vi "Joystick Get Values.vi"(8 "error in (no error)":errorcluster, 11 "Joystick":T1) -> (0 "error out":errorcluster, 1 "Buttons":bool[](array[boolean]), 2 "Axes":dbl[](array[numeric]), 3 "Joystick":T1, 4 "POVs":u8[](array[numeric]), 5 "Touchpads":T2(array[cluster]))   [LabVIEW 2026, in "MrcLib.lvlib"]
doc: "Returns button and scaled axis information for a joystick that you specify."
uses:
  MrcLib.lvlib
  <vilib>/Rock Robotics/WPI/Joystick/WPI_JoystickDeviceEnum.ctl
panel:
  in  "Scaler":i16=32767
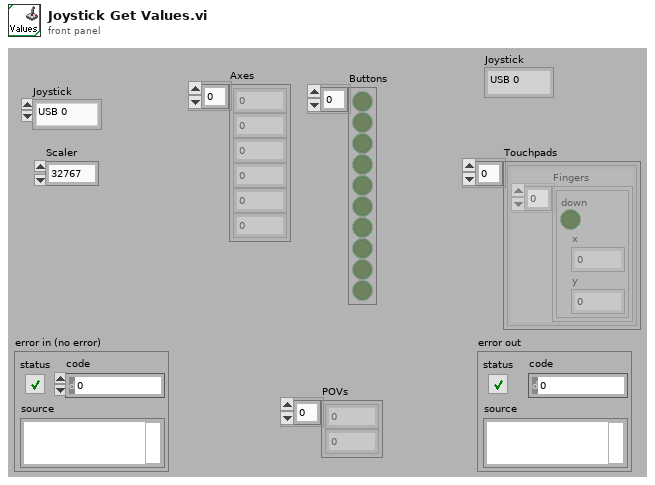
[diagram p1: front panel]
types:
  T1 = typedef "WPI_JoystickDeviceEnum.ctl" = enum16{"USB 0", "USB 1", "USB 2", "USB 3", "USB 4", "USB 5"}
  T2 = cluster{"Fingers":cluster{"down":bool, "x":u16, "y":u16}[]}[]
  T3 = cluster{cluster{"down":bool, "x":u16, "y":u16}[]}
  T4 = typedef "MrcLib.lvlib/MRC_Joysticks.ctl" = cluster{"count":u8, "dummy":cluster{i8, i8, i8, i8, i8, i8, i8}, "joystick 0":cluster{"availablePovs":u8, "povs":cluster{"pov 0":u8, "pov 1":u8, "pov 2":u8, "pov 3":u8, "pov 4":u8, "pov 5":u8, "pov 6":u8, "pov 7":u8}, "availableAxes":u16, "axes":cluster{"axis 0":i16, "axis 1":i16, "axis 2":i16, "axis 3":i16, "axis 4":i16, "axis 5":i16, "axis 6":i16, "axis 7":i16, "axis 8":i16, "axis 9":i16, "axis 10":i16, "axis 11":i16}, "availableButtons":u64, "buttons":u64, "touchPads":cluster{"touchPadCount":u8, "touchpad 1":cluster{"count":u8, "finger 1":cluster{"down":u8, "x":u16, "y":u16}, "finger 2":cluster{"down":u8, "x":u16, "y":u16}}, "touchpad 2":cluster{"count":u8, "finger 1":cluster{"down":u8, "x":u16, "y":u16}, "finger 2":cluster{"down":u8, "x":u16, "y":u16}}}}, "joystick 1":cluster{"availablePovs":u8, "povs":cluster{"pov 0":u8, "pov 1":u8, "pov 2":u8, "pov 3":u8, "pov 4":u8, "pov 5":u8, "pov 6":u8, "pov 7":u8}, "availableAxes":u16, "axes":cluster{"axis 0":i16, "axis 1":i16, "axis 2":i16, "axis 3":i16, "axis 4":i16, "axis 5":i16, "axis 6":i16, "axis 7":i16, "axis 8":i16, "axis 9":i16, "axis 10":i16, "axis 11":i16}, "availableButtons":u64, "buttons":u64, "touchPads":cluster{"touchPadCount":u8, "touchpad 1":cluster{"count":u8, "finger 1":cluster{"down":u8, "x":u16, "y":u16}, "finger 2":cluster{"down":u8, "x":u16, "y":u16}}, "touchpad 2":cluster{"count":u8, "finger 1":cluster{"down":u8, "x":u16, "y":u16}, "finger 2":cluster{"down":u8, "x":u16, "y":u16}}}}, "joystick 2":cluster{"availablePovs":u8, "povs":cluster{"pov 0":u8, "pov 1":u8, "pov 2":u8, "pov 3":u8, "pov 4":u8, "pov 5":u8, "pov 6":u8, "pov 7":u8}, "availableAxes":u16, "axes":cluster{"axis 0":i16, "axis 1":i16, "axis 2":i16, "axis 3":i16, "axis 4":i16, "axis 5":i16, "axis 6":i16, "axis 7":i16, "axis 8":i16, "axis 9":i16, "axis 10":i16, "axis 11":i16}, "availableButtons":u64, "buttons":u64, "touchPads":cluster{"touchPadCount":u8, "touchpad 1":cluster{"count":u8, "finger 1":cluster{"down":u8, "x":u16, "y":u16}, "finger 2":cluster{"down":u8, "x":u16, "y":u16}}, "touchpad 2":cluster{"count":u8, "finger 1":cluster{"down":u8, "x":u16, "y":u16}, "finger 2":cluster{"down":u8, "x":u16, "y":u16}}}}, "joystick 3":cluster{"availablePovs":u8, "povs":cluster{"pov 0":u8, "pov 1":u8, "pov 2":u8, "pov 3":u8, "pov 4":u8, "pov 5":u8, "pov 6":u8, "pov 7":u8}, "availableAxes":u16, "axes":cluster{"axis 0":i16, "axis 1":i16, "axis 2":i16, "axis 3":i16, "axis 4":i16, "axis 5":i16, "axis 6":i16, "axis 7":i16, "axis 8":i16, "axis 9":i16, "axis 10":i16, "axis 11":i16}, "availableButtons":u64, "buttons":u64, "touchPads":cluster{"touchPadCount":u8, "touchpad 1":cluster{"count":u8, "finger 1":cluster{"down":u8, "x":u16, "y":u16}, "finger 2":cluster{"down":u8, "x":u16, "y":u16}}, "touchpad 2":cluster{"count":u8, "finger 1":cluster{"down":u8, "x":u16, "y":u16}, "finger 2":cluster{"down":u8, "x":u16, "y":u16}}}}, "joystick 4":cluster{"availablePovs":u8, "povs":cluster{"pov 0":u8, "pov 1":u8, "pov 2":u8, "pov 3":u8, "pov 4":u8, "pov 5":u8, "pov 6":u8, "pov 7":u8}, "availableAxes":u16, "axes":cluster{"axis 0":i16, "axis 1":i16, "axis 2":i16, "axis 3":i16, "axis 4":i16, "axis 5":i16, "axis 6":i16, "axis 7":i16, "axis 8":i16, "axis 9":i16, "axis 10":i16, "axis 11":i16}, "availableButtons":u64, "buttons":u64, "touchPads":cluster{"touchPadCount":u8, "touchpad 1":cluster{"count":u8, "finger 1":cluster{"down":u8, "x":u16, "y":u16}, "finger 2":cluster{"down":u8, "x":u16, "y":u16}}, "touchpad 2":cluster{"count":u8, "finger 1":cluster{"down":u8, "x":u16, "y":u16}, "finger 2":cluster{"down":u8, "x":u16, "y":u16}}}}, "joystick 5":cluster{"availablePovs":u8, "povs":cluster{"pov 0":u8, "pov 1":u8, "pov 2":u8, "pov 3":u8, "pov 4":u8, "pov 5":u8, "pov 6":u8, "pov 7":u8}, "availableAxes":u16, "axes":cluster{"axis 0":i16, "axis 1":i16, "axis 2":i16, "axis 3":i16, "axis 4":i16, "axis 5":i16, "axis 6":i16, "axis 7":i16, "axis 8":i16, "axis 9":i16, "axis 10":i16, "axis 11":i16}, "availableButtons":u64, "buttons":u64, "touchPads":cluster{"touchPadCount":u8, "touchpad 1":cluster{"count":u8, "finger 1":cluster{"down":u8, "x":u16, "y":u16}, "finger 2":cluster{"down":u8, "x":u16, "y":u16}}, "touchpad 2":cluster{"count":u8, "finger 1":cluster{"down":u8, "x":u16, "y":u16}, "finger 2":cluster{"down":u8, "x":u16, "y":u16}}}}}
  T5 = cluster{"availablePovs":u8, "povs":cluster{"pov 0":u8, "pov 1":u8, "pov 2":u8, "pov 3":u8, "pov 4":u8, "pov 5":u8, "pov 6":u8, "pov 7":u8}, "availableAxes":u16, "axes":cluster{"axis 0":i16, "axis 1":i16, "axis 2":i16, "axis 3":i16, "axis 4":i16, "axis 5":i16, "axis 6":i16, "axis 7":i16, "axis 8":i16, "axis 9":i16, "axis 10":i16, "axis 11":i16}, "availableButtons":u64, "buttons":u64, "touchPads":cluster{"touchPadCount":u8, "touchpad 1":cluster{"count":u8, "finger 1":cluster{"down":u8, "x":u16, "y":u16}, "finger 2":cluster{"down":u8, "x":u16, "y":u16}}, "touchpad 2":cluster{"count":u8, "finger 1":cluster{"down":u8, "x":u16, "y":u16}, "finger 2":cluster{"down":u8, "x":u16, "y":u16}}}}
  T6 = cluster{"pov 0":u8, "pov 1":u8, "pov 2":u8, "pov 3":u8, "pov 4":u8, "pov 5":u8, "pov 6":u8, "pov 7":u8}
  T7 = cluster{"axis 0":i16, "axis 1":i16, "axis 2":i16, "axis 3":i16, "axis 4":i16, "axis 5":i16, "axis 6":i16, "axis 7":i16, "axis 8":i16, "axis 9":i16, "axis 10":i16, "axis 11":i16}
  T8 = cluster{"touchPadCount":u8, "touchpad 1":cluster{"count":u8, "finger 1":cluster{"down":u8, "x":u16, "y":u16}, "finger 2":cluster{"down":u8, "x":u16, "y":u16}}, "touchpad 2":cluster{"count":u8, "finger 1":cluster{"down":u8, "x":u16, "y":u16}, "finger 2":cluster{"down":u8, "x":u16, "y":u16}}}
  T9 = cluster{"count":u8, "finger 1":cluster{"down":u8, "x":u16, "y":u16}, "finger 2":cluster{"down":u8, "x":u16, "y":u16}}
  T10 = cluster{"count":u8, "finger 1":cluster{"down":u8, "x":u16, "y":u16}, "finger 2":cluster{"down":u8, "x":u16, "y":u16}}[]
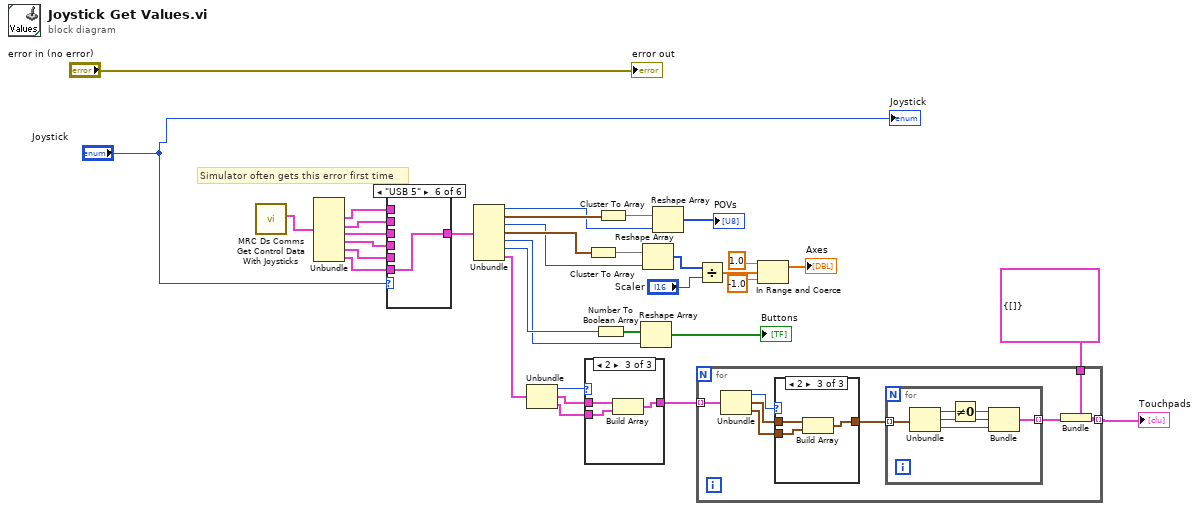
[diagram p0: block diagram]
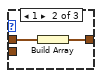
[diagram p3: hidden frame]
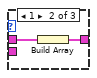
[diagram p5: hidden frame]
diagram:
  # "Simulator often gets this error first time"
  n1 = call "MRC Ds Comms Get Control Data With Joysticks.vi"() -> ("joystickData out"=w30:T4)  [unwired: 9 in, 2 out]
  n2 = Unbundle(w30) -> ("joystick 0"=w29:T5, "joystick 1"=w28:T5, "joystick 2"=w27:T5, "joystick 3"=w26:T5, "joystick 4"=w25:T5, "joystick 5"=w24:T5)  [unwired: 2 out]
  n3 = case shown="\"USB 5\"" "Joystick" {
    tunnel: [w35 w36 w37 w38 w39 w40] -> w23
    tunnel: w29 -> [w35 _ _ _ _ _]
    tunnel: w28 -> [_ w36 _ _ _ _]
    tunnel: w27 -> [_ _ w37 _ _ _]
    tunnel: w26 -> [_ _ _ w38 _ _]
    tunnel: w25 -> [_ _ _ _ w39 _]
    tunnel: w24 -> [_ _ _ _ _ w40]
    frame "USB 0", Default {
    }
    frame "USB 1" {
    }
    frame "USB 2" {
    }
    frame "USB 3" {
    }
    frame "USB 4" {
    }
    frame "USB 5" {
    }
  }
  n4 = Unbundle(w23) -> ("availablePovs"=w20:u8, "povs"=w22:T6, "availableAxes"=w16:u16, "axes"=w17:T7, "availableButtons"=w11:u64, "buttons"=w12:u64, "touchPads"=w9:T8)
  n5 = Unbundle(w9) -> ("touchPadCount"=w8:u8, "touchpad 1"=w7:T9, "touchpad 2"=w6:T9)
  n6 = case shown="2" w8 {
    tunnel: w7 -> [_ w42 w45]
    tunnel: w6 -> [_ _ w44]
    tunnel: [_ w41 w43] -> w5
    frame 0, Default {
    }
    frame 1 {
      n7 = Build Array(w42) -> (w41:T10)
    }
    frame 2 {
      n8 = Build Array(w45, w44) -> (w43:T10)
    }
  }
  n9 = Cluster To Array(cluster=w17) -> (array=w18:i16[])
  n10 = Number To Boolean Array(number=w12) -> (Boolean array=w13:bool[])
  n11 = Cluster To Array(cluster=w22) -> (array=w21:u8[])
  n12 = Reshape Array(w13, w11) -> (→"Buttons":bool[])
  n13 = Reshape Array(w18, w16) -> (w15:i16[])
  n14 = Reshape Array(w21, w20) -> (→"POVs":u8[])
  n15 = Divide(x=w15, y="Scaler") -> (x/y=w34:dbl[])
  n16 = for {
    tunnel: w5 -> [w53] mode=indexing
    tunnel: [w47] -> w3 mode=indexing
    tunnel: T3 {[]} -> [w46]
    n17 = Unbundle(w53) -> ("count"=w52:u8, "finger 1"=w51:cluster{"down":u8, "x":u16, "y":u16}, "finger 2"=w50:cluster{"down":u8, "x":u16, "y":u16})
    n18 = case shown="2" w52 {
      tunnel: w51 -> [_ w61 w64]
      tunnel: w50 -> [_ _ w63]
      tunnel: [_ w60 w62] -> w49
      frame 0, Default {
      }
      frame 1 {
        n19 = Build Array(w61) -> (w60:cluster{"down":u8, "x":u16, "y":u16}[])
      }
      frame 2 {
        n20 = Build Array(w64, w63) -> (w62:cluster{"down":u8, "x":u16, "y":u16}[])
      }
    }
    n21 = for {
      tunnel: w49 -> [w59] mode=indexing
      tunnel: [w54] -> w48 mode=indexing
      n22 = Unbundle(w59) -> ("down"=w58:u8, "x"=w56:u16, "y"=w55:u16)
      n23 = Not Equal To 0?(x=w58) -> (x != 0?=w57:bool)
      n24 = Bundle(w57, "x"=w56, "y"=w55) -> (w54:cluster{bool, "x":u16, "y":u16})  [unwired: 1 in]
    }
    n25 = Bundle(cluster=w46, w48) -> (w47:T3)
  }
  "Touchpads" <- w3
  n26 = In Range and Coerce(upper limit=1.0, x=w34, lower limit=-1.0) -> (coerced(x)=→"Axes":dbl[])  [unwired: 1 out]
  "error out" <- "error in (no error)"
  "Joystick" <- "Joystick"
